vi "main.vi"() -> ()   [LabVIEW 2020]
uses:
  Global 1.vi
  <extravilib>/ChannelInstances/Lossy Stream-a[.,.](dbl)/Instantiate.vi
  <extravilib>/ChannelInstances/Stream-a[.](dbl)/Instantiate.vi
  <extravilib>/ChannelInstances/Lossy Stream-a[.](dbl)/Instantiate.vi
  <extravilib>/ChannelInstances/Lossy Stream-a[.](u8)/Instantiate.vi
  <vilib>/MakerHub/LINX/Public/Utilities/Open Local.vi
  <extravilib>/ChannelInstances/Stream-a[.,.](dbl)/Instantiate.vi
  <vilib>/MakerHub/LINX/LMH-LINX.lvlib
panel:
  out "Main Loop":i32
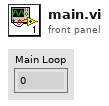
[diagram p1: front panel]
types:
  T1 = enum16{"open", "open or create", "create or replace", "create", "open (read-only)"}
  T2 = typedef "LMH-LINX.lvlib/LINX Ref.ctl" = cluster{"IO":T3, "Interface":T4, "LINX Device Config":T5}
  T3 = typedef "LMH-LINX.lvlib/Platform.ctl" = enum16{"Remote", "Local"}
  T4 = typedef "LMH-LINX.lvlib/Interface.ctl" = enum16{"Serial", "TCP"}
  T5 = typedef "LMH-LINX.lvlib/Device.lvlib/LINX Device Config.ctl" = cluster{"Interface":T4, "COM Port":refnum<visa-resource-name>, "TCP Configuration":T6, "Device Family":u8, "Device ID":u8, "Device Name":string, "TCP Ref":refnum<k5>, "Channels":T7}
  T6 = typedef "LMH-LINX.lvlib/Device.lvlib/TCP Config.ctl" = cluster{"IP Address":string, "Port":u16}
  T7 = typedef "LMH-LINX.lvlib/Channels.ctl" = cluster{"DI":u8[], "DO":u8[], "AI":u8[], "AO":u8[], "PWM":u8[], "QE":u8[], "UART":u8[], "I2C 2":u8[], "SPI":u8[], "CAN":u8[], "Servo":u8[], "AI Ref (V)":dbl, "AI Resolution (Bits)":u8, "AO Ref (V)":dbl, "AO Resolution (Bits)":u8}
  T8 = typedef "Lossy Stream-a[.](u8).lvlib/)Channel.ctl" = refnum<queue>
  T9 = typedef "Lossy Stream-a[.](dbl).lvlib/)Channel.ctl" = refnum<queue>
  T10 = typedef "Stream-a[.](dbl).lvlib/)Channel.ctl" = refnum<queue>
  T11 = typedef "Lossy Stream-a[.,.](dbl).lvlib/)Channel.ctl" = refnum<queue>
  T12 = cluster{"error out":errorcluster, "Error Out":errorcluster, "error out":errorcluster, "error out":errorcluster, "error out":errorcluster}
  T13 = typedef "Stream-a[.,.](dbl).lvlib/)Channel.ctl" = refnum<queue>
  T14 = cluster{"error out":errorcluster, "error out":errorcluster, "Error Out":errorcluster, "error out":errorcluster, "error out":errorcluster, "error out":errorcluster, "error out":errorcluster, "error out":errorcluster}
  T15 = cluster{"Hyperparameters":cluster{"Kernel Type":string, "Alpha (idx)":dbl[][], "Training (idx)":dbl[][], "Label (idx)":dbl[][], "w":dbl[][], "b":dbl, "Performance":cluster{"True Negatives":i32, "False Negatives":i32, "True Positives":i32, "False Positives":i32, "Accuracy":dbl, "F Score":dbl, "Precision":dbl}, "gamma_opt":dbl, "C_opt":dbl}, i32, dbl, "Data Buffer":dbl[][]}
  T16 = cluster{"Kernel Type":string, "Alpha (idx)":dbl[][], "Training (idx)":dbl[][], "Label (idx)":dbl[][], "w":dbl[][], "b":dbl, "Performance":cluster{"True Negatives":i32, "False Negatives":i32, "True Positives":i32, "False Positives":i32, "Accuracy":dbl, "F Score":dbl, "Precision":dbl}, "gamma_opt":dbl, "C_opt":dbl}
  T17 = cluster{"error out":errorcluster, "error out":errorcluster, "Error Out":errorcluster, "error out":errorcluster, "error out":errorcluster, "error out":errorcluster, "error out":errorcluster, "error out":errorcluster, "error out":errorcluster, "error out":errorcluster}
  T18 = cluster{"Kernel Type":string, "Alpha (idx)":dbl[][], "Training (idx)":dbl[][], "Label (idx)":dbl[][], "w":dbl[][], "b":dbl, "Performance":cluster{"True Negatives":i32, "False Negatives":i32, "True Positives":i32, "False Positives":i32, "Accuracy":dbl, "F Score":dbl, "F Score 2":dbl}, "gamma_opt":dbl, "C_opt":dbl}
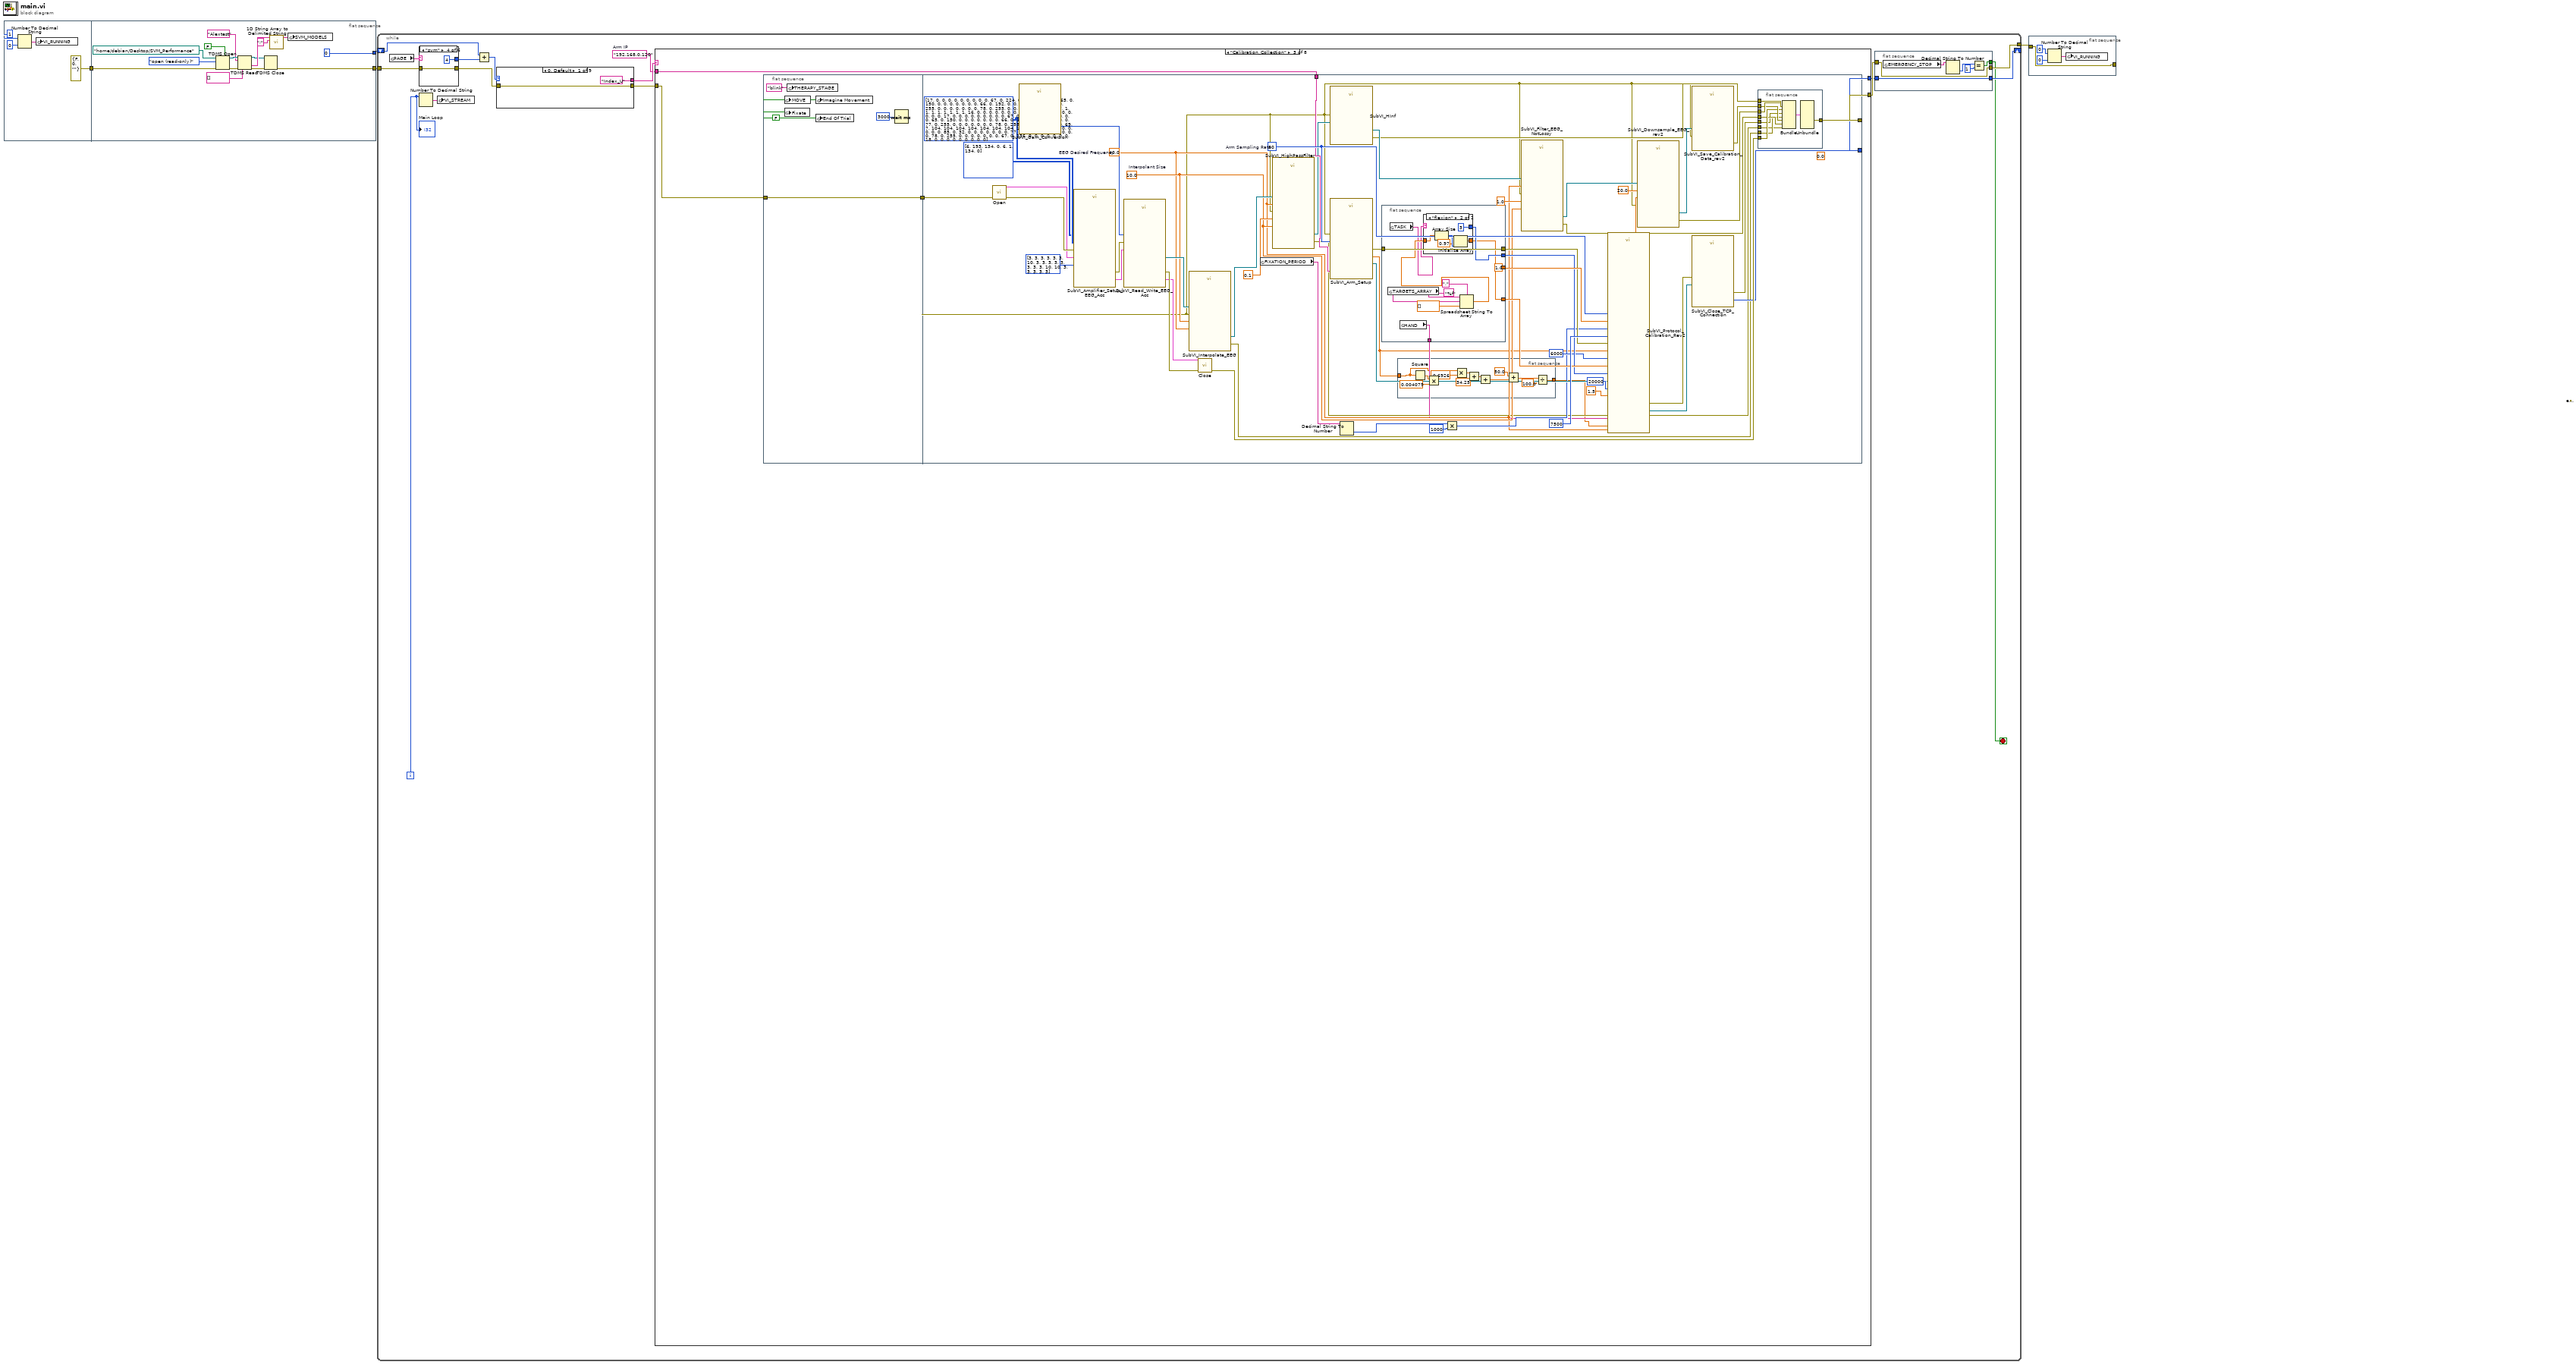
[diagram p0: block diagram]
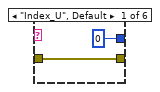
[diagram p2: hidden frame]
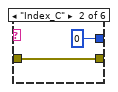
[diagram p3: hidden frame]
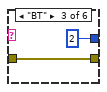
[diagram p4: hidden frame]
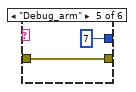
[diagram p5: hidden frame]
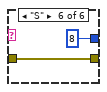
[diagram p6: hidden frame]
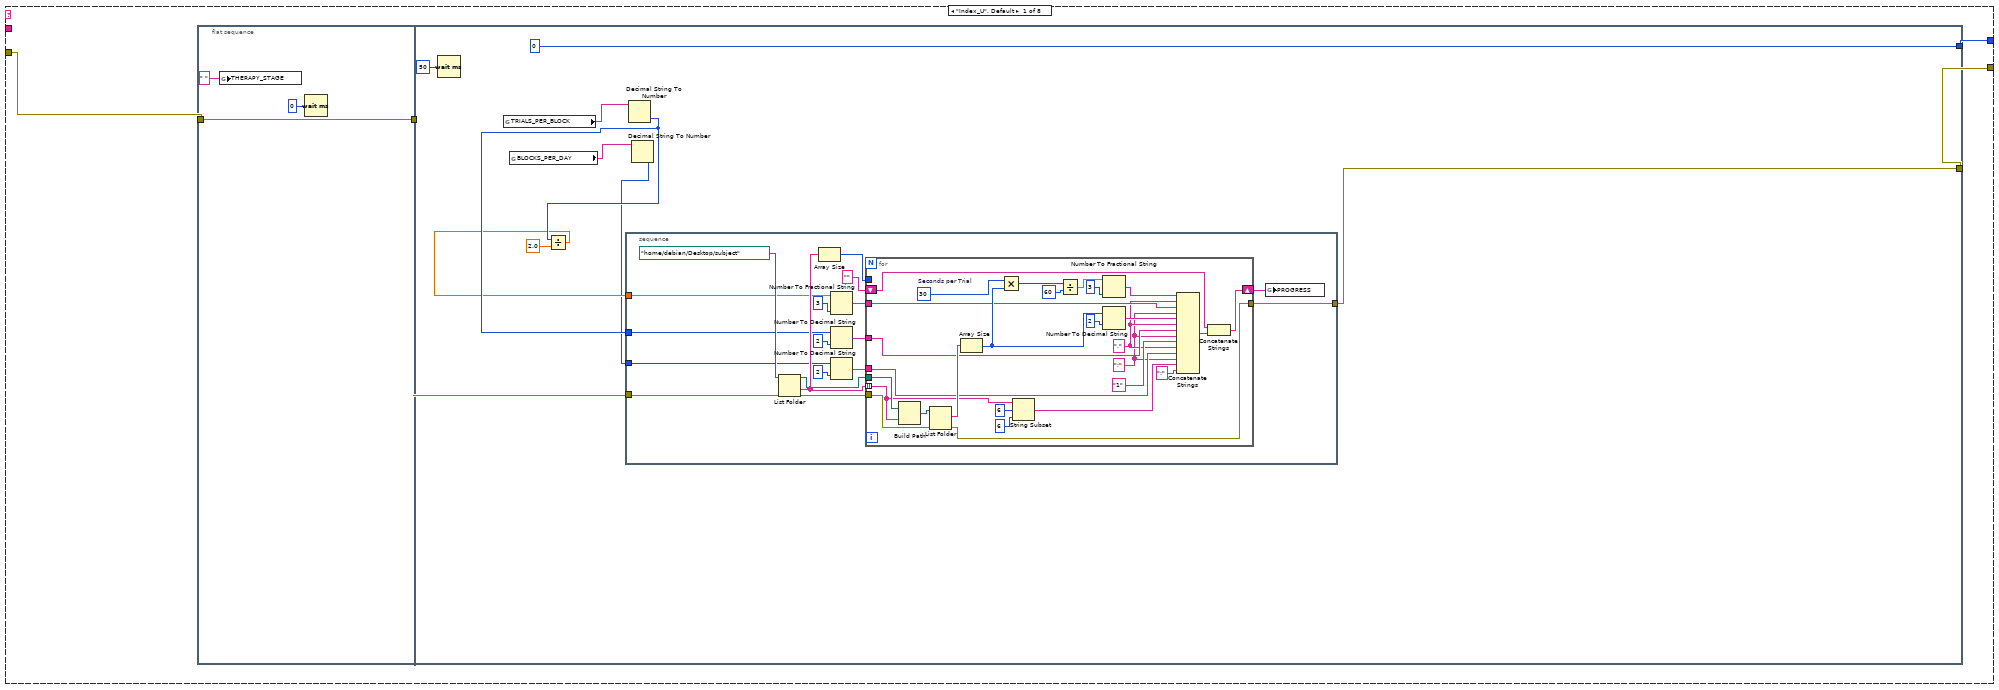
[diagram p7: hidden frame]
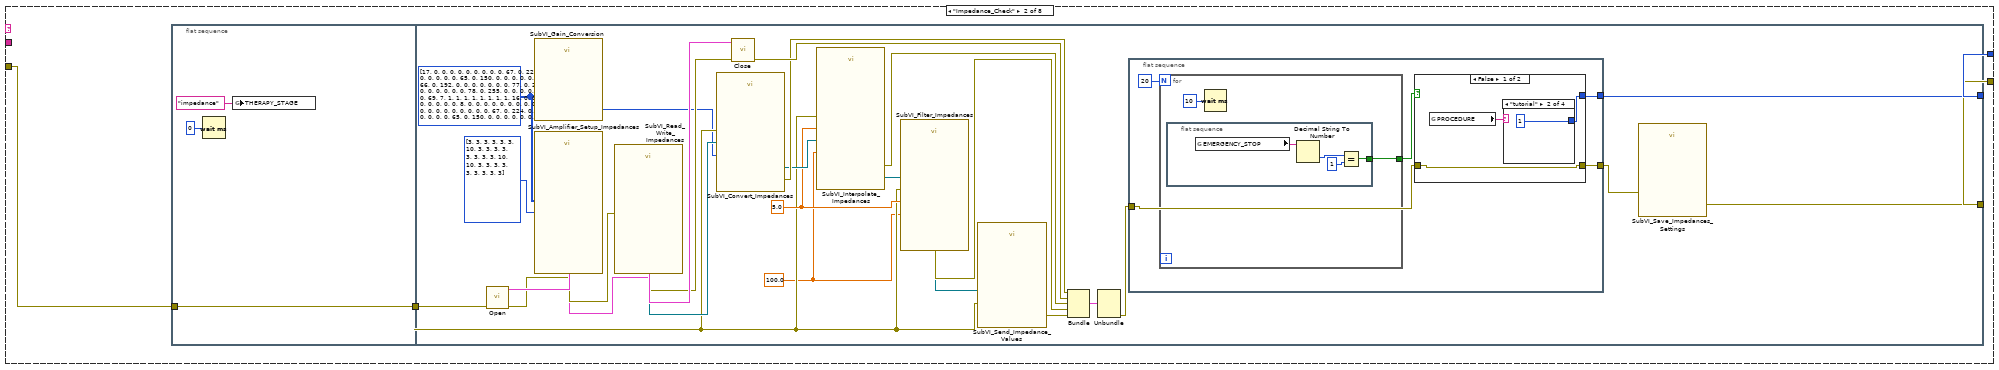
[diagram p8: hidden frame]
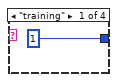
[diagram p9: hidden frame]
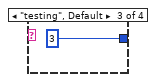
[diagram p10: hidden frame]
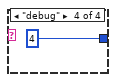
[diagram p11: hidden frame]
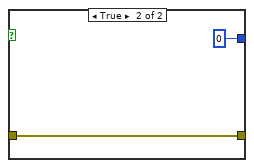
[diagram p12: hidden frame]
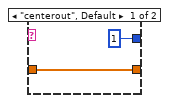
[diagram p13: hidden frame]
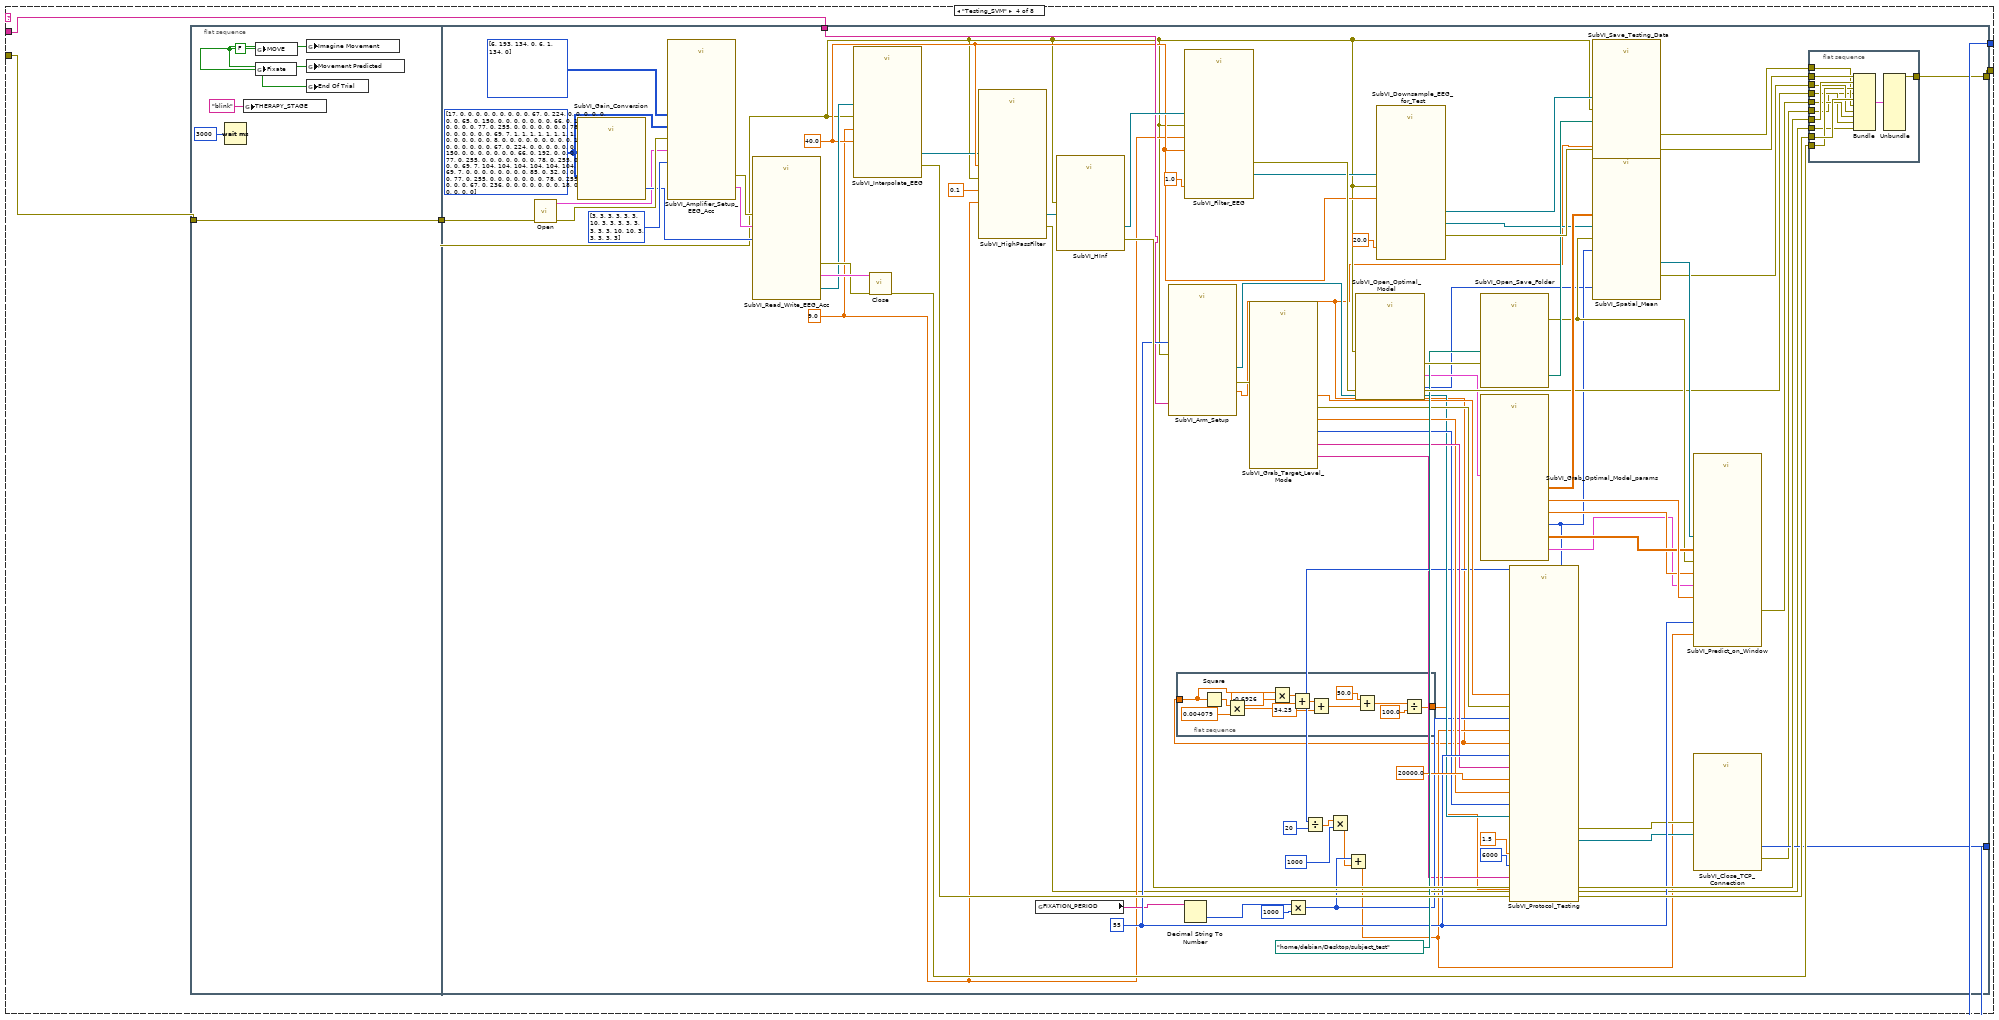
[diagram p14: hidden frame]
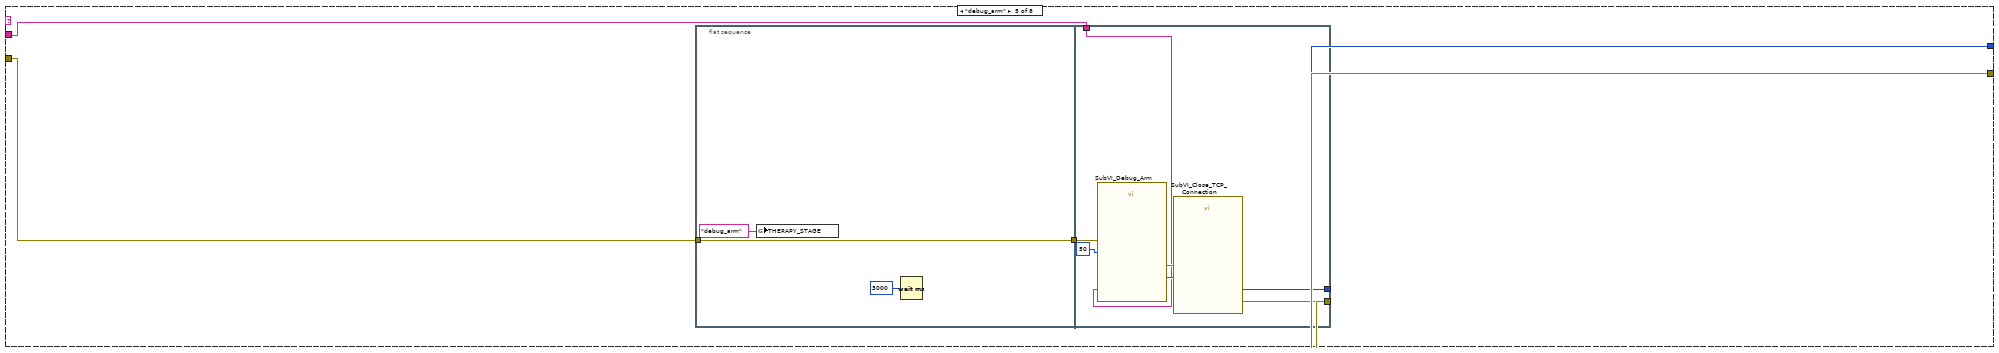
[diagram p15: hidden frame]
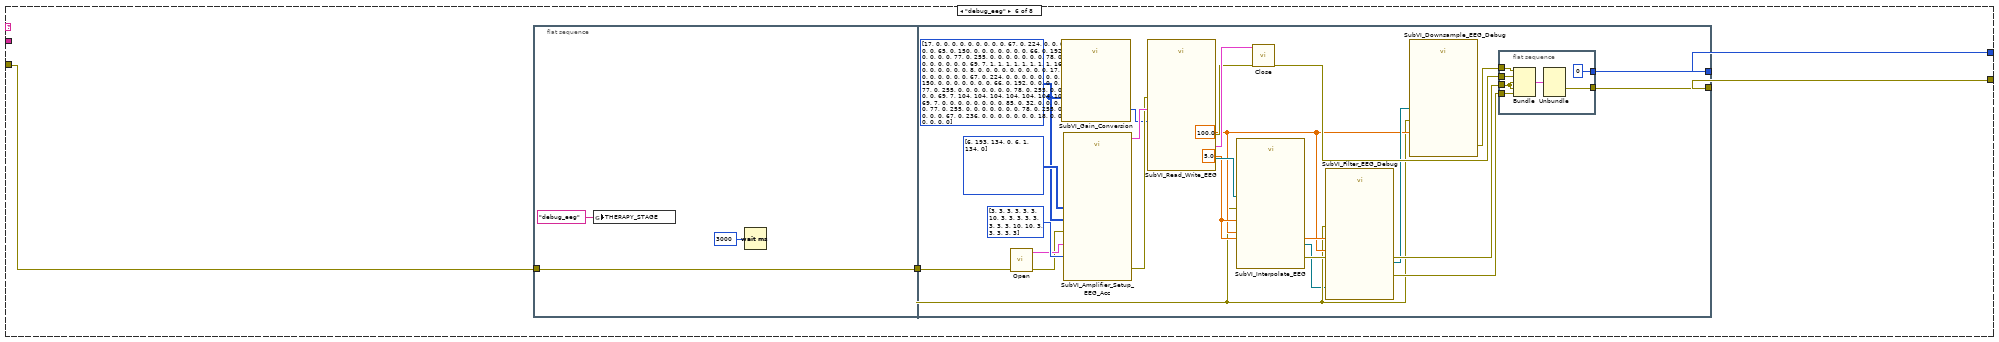
[diagram p16: hidden frame]
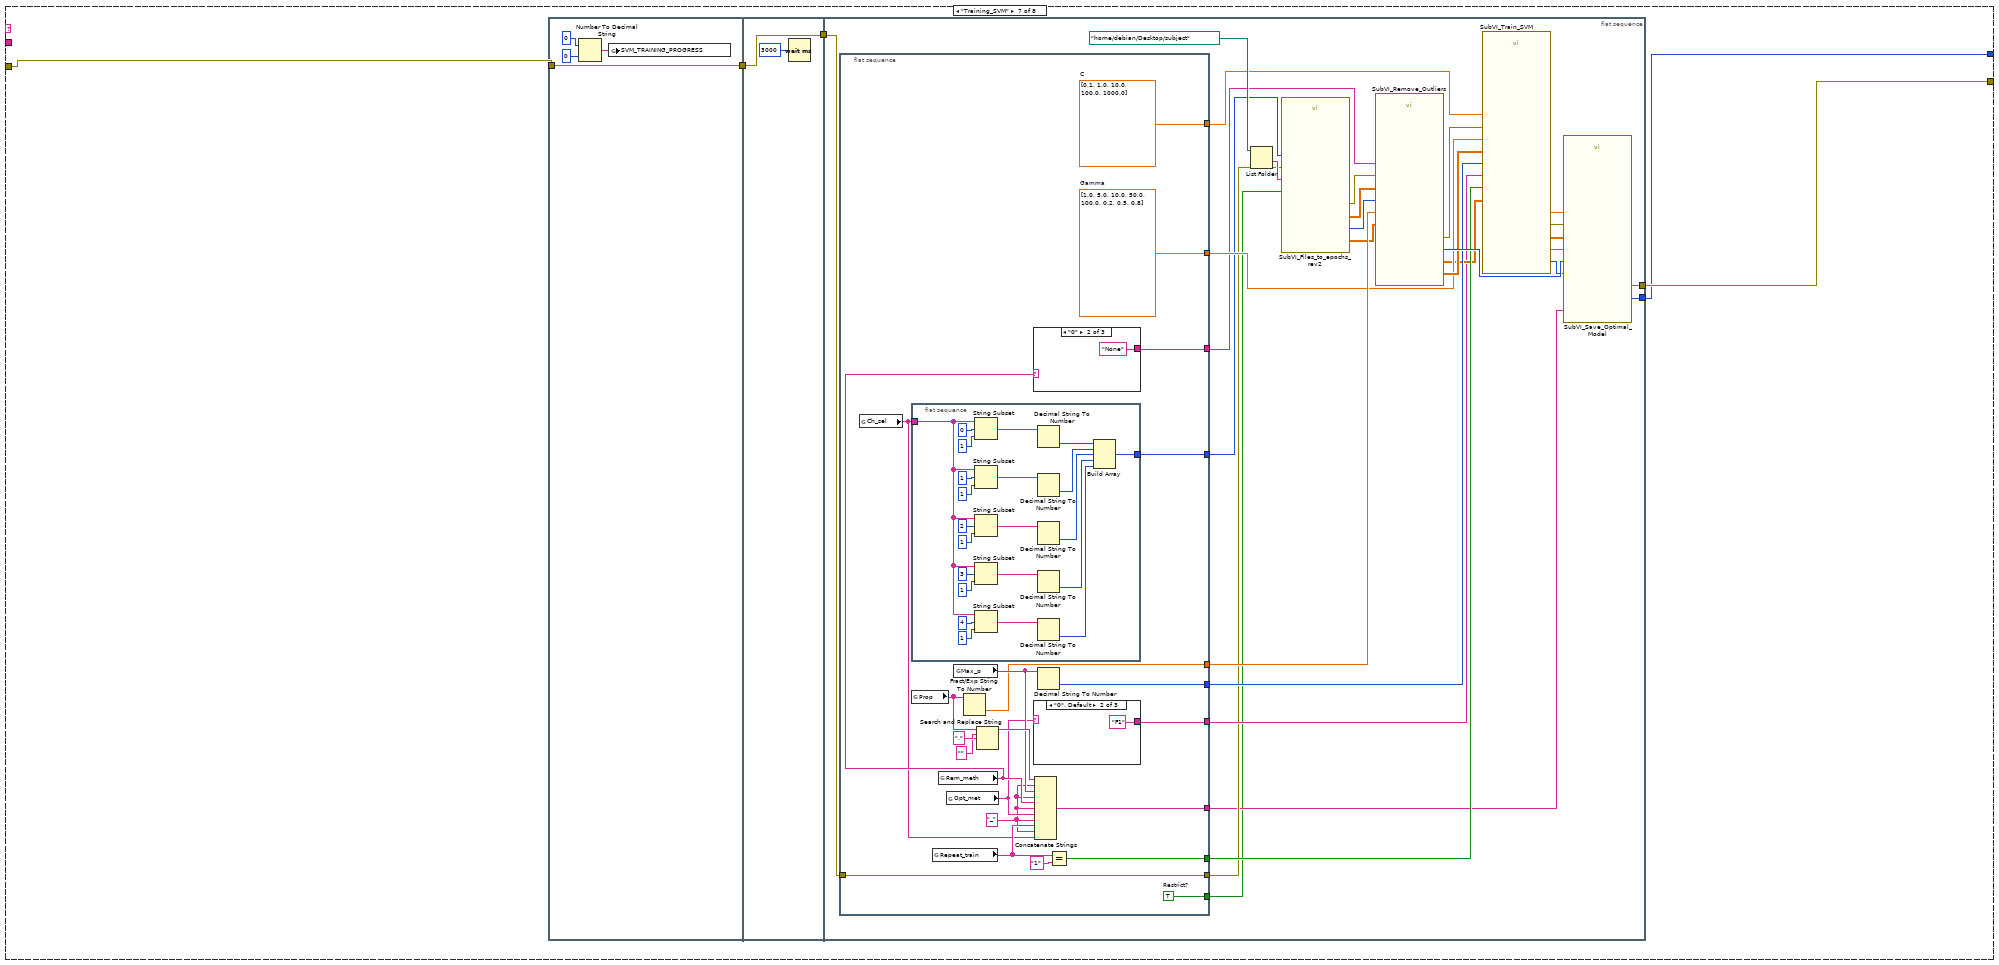
[diagram p17: hidden frame]
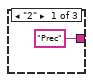
[diagram p18: hidden frame]
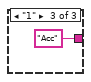
[diagram p19: hidden frame]
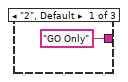
[diagram p20: hidden frame]
diagram:
  (unwired) errorcluster {"status"=FALSE, "code"=0, "source"=""} ("error in (no error)")
  n1 = flat-sequence {
    tunnel: [errorcluster {"status"=FALSE, "code"=0, "source"=""} ("error in (no error)")] -> w2
    tunnel: w2 -> [w13]
    tunnel: [w10] -> w4
    tunnel: [0] -> w1
    frame #0 {
      n2 = Number To Decimal String(number=1, width (-)=i16 0) -> (decimal integer string=w8:string)
      n3 = global write "Global 1.vi" "VI_RUNNING"(w8) -> ()
    }
    frame #1 {
      n4 = TDMS Open(5:FALSE ("create index file? (T)"), 8:w13, 10:T1."open (read-only)" ("operation (0:open)"), 11:path "/home/debian/Desktop/SVM_Performance" ("base path")) -> (0:w18:errorcluster, 3:w19:refnum<k34>)  [unwired: 3 in]
      n5 = TDMS Read(0:w19, 5:"Alextest" ("group name in (Untitled)"), 11:w18, 12:string[] []) -> (4:w21:refnum<k34>, 10:w22:string[], 15:w20:errorcluster)  [unwired: 4 in, 3 out]
      n6 = TDMS Close(8:w20, 11:w21) -> (0:w10:errorcluster)  [unwired: 1 out]
      n7 = call <vilib>:"1D String Array to Delimited String.vi"("delimiter"=";", "string array"=w22) -> ("delimited string"=w23:string)  [unwired: 9 in]
      n8 = global write "Global 1.vi" "SVM_MODELS"(w23) -> ()
    }
  }
  n9 = while {
    tunnel: w4 -> [w35]
    tunnel: [w27] -> w3
    shift-right: [w28] -> _
    shift-left: w1 -> [w33]
    i -> [w31]
    stop <- w25 stop-if-true
    w24 = "192.168.0.120"  # Arm IP
    n10 = global read "Global 1.vi" "PAGE"() -> (w32:string)
    n11 = case shown="\"svm\"" w32 {
      tunnel: [0 0 2 4 7 8] -> w39
      tunnel: [w46 w48 w50 w53 w54 w56] -> w36
      tunnel: w35 -> [w46 w48 w50 w53 w54 w56]
      frame "Index_U", Default {
      }
      frame "Index_C" {
      }
      frame "BT" {
      }
      frame "svm" {
      }
      frame "Debug_arm" {
      }
      frame "S" {
      }
    }
    n12 = Number To Decimal String(number=w31) -> (decimal integer string=w30:string)  [unwired: 1 in]
    n13 = global write "Global 1.vi" "VI_STREAM"(w30) -> ()
    n14 = Add(x=w33, y=w39) -> (x+y=w38:i32)
    n15 = case shown="0, Default" w38 {
      tunnel: ["Index_U" "Index_C" "Impedance_Check" "Calibration_Collection" "Training_SVM" "Testing_SVM" "debug_eeg" "debug_arm" "Survey"] -> w37
      tunnel: w36 -> [w537 w539 w542 w545 w548 w551 w554 w557 w559]
      tunnel: [w537 w539 w542 w545 w548 w551 w554 w557 w559] -> w34
      frame 0, Default {
      }
      frame 1 {
      }
      frame 2 {
        n16 = global write "Global 1.vi" "THERAPY_STAGE"("impedance" ("THERAPY_STAGE")) -> ()
      }
      frame 3 {
        n17 = global write "Global 1.vi" "THERAPY_STAGE"(" " ("THERAPY_STAGE")) -> ()
      }
      frame 4 {
        n18 = global write "Global 1.vi" "THERAPY_STAGE"(" " ("THERAPY_STAGE")) -> ()
      }
      frame 5 {
        n19 = global write "Global 1.vi" "THERAPY_STAGE"(" " ("THERAPY_STAGE")) -> ()
      }
      frame 6 {
        n20 = global write "Global 1.vi" "THERAPY_STAGE"(" " ("THERAPY_STAGE")) -> ()
      }
      frame 7 {
        n21 = global write "Global 1.vi" "THERAPY_STAGE"(" " ("THERAPY_STAGE")) -> ()
      }
      frame 8 {
      }
    }
    n22 = case shown="\"Calibration_Collection\"" w37 {
      tunnel: [w59 w123 w177 w281 w387 w402 w439 w528] -> w26
      tunnel: w34 -> [w61 w124 w176 w279 w389 w401 w438 w530]
      tunnel: [w60 w121 w178 w280 w388 w403 w440 w529] -> w29
      tunnel: w24 -> [_ _ w175 w277 w385 _ _ _]
      frame "Index_U", Default {
        n23 = flat-sequence {
          tunnel: w61 -> [w64]
          tunnel: [w64] -> w58
          tunnel: [w71] -> w60
          tunnel: [0 ("Tab Select")] -> w59
          tunnel: w58 -> [w72]
          frame #0 {
            n24 = global write "Global 1.vi" "THERAPY_STAGE"(" " ("THERAPY_STAGE")) -> ()
            n25 = Wait (ms)(milliseconds to wait=u32 0) -> ()  [unwired: 1 out]
          }
          frame #1 {
            n26 = Wait (ms)(milliseconds to wait=u32 50) -> ()  [unwired: 1 out]
            n27 = global read "Global 1.vi" "TRIALS_PER_BLOCK"() -> (w69:string)
            n28 = global read "Global 1.vi" "BLOCKS_PER_DAY"() -> (w70:string)
            n29 = Decimal String To Number(string=w69) -> (number=w67:i32)  [unwired: 2 in, 1 out]
            n30 = Divide(x=w67, y=2.0) -> (x/y=w66:dbl)
            n31 = Decimal String To Number(string=w70) -> (number=w65:i32)  [unwired: 2 in, 1 out]
            n32 = stacked-sequence {
              tunnel: w72 -> [w92]
              tunnel: w66 -> [w80]
              tunnel: w65 -> [w82]
              tunnel: w67 -> [w81]
              tunnel: [w75] -> w71
              frame #0 {
                n33 = List Folder(path=path "/home/debian/Desktop/subject" ("base path"), error in=w92) -> (path out=w90:path, folder names=w88:string[], error out=w89:errorcluster)  [unwired: 2 in, 1 out]
                n34 = Array Size(array=w88) -> (size(s)=w87:i32)
                n35 = Number To Fractional String(number=w80, precision (6)=i16 3) -> (F-format string=w79:string)  [unwired: 2 in]
                n36 = Number To Decimal String(number=w81, width (-)=i16 2) -> (decimal integer string=w78:string)
                n37 = Number To Decimal String(number=w82, width (-)=i16 2) -> (decimal integer string=w77:string)
                n38 = for {
                  tunnel: w88 -> [w96] mode=indexing
                  tunnel: w90 -> [w120]
                  tunnel: w89 -> [w118]
                  tunnel: [w117] -> w75
                  tunnel: w87 -> [_]
                  shift-right: [w115] -> w76
                  shift-left: "" -> [w116]
                  tunnel: w79 -> [w104]
                  tunnel: w78 -> [w102]
                  tunnel: w77 -> [w99]
                  w98 = ";" ("string")
                  w100 = "," ("string")
                  w112 = 30  # Seconds per Trial
                  n39 = Build Path(base path=w120, name or relative path=w96) -> (appended path=w119:path)
                  n40 = List Folder(path=w119, error in=w118) -> (filenames=w114:string[], error out=w117:errorcluster)  [unwired: 2 in, 2 out]
                  n41 = Array Size(array=w114) -> (size(s)=w107:i32)
                  n42 = Multiply(x=w112, y=w107) -> (x*y=w111:i32)
                  n43 = String Subset(string=w96, offset (0)=6, length (rest)=6 ("length (rest)")) -> (substring=w93:string)
                  n44 = Divide(x=w111, y=60) -> (x/y=w108:dbl)
                  n45 = Number To Fractional String(number=w108, precision (6)=i16 3) -> (F-format string=w106:string)  [unwired: 2 in]
                  n46 = Number To Decimal String(number=w107, width (-)=i16 2) -> (decimal integer string=w103:string)
                  n47 = Concatenate Strings(w106, w100, w104, w98, w103, w100, w102, w98, "1" ("string"), w100, w99, w98, w93, ":" ("string")) -> (w105:string)
                  n48 = Concatenate Strings(w116, w105) -> (w115:string)
                }
                n49 = global write "Global 1.vi" "PROGRESS"(w76) -> ()
              }
            }
          }
        }
      }
      frame "Impedance_Check" {
        n50 = flat-sequence {
          tunnel: w124 -> [w127]
          tunnel: [w127] -> w122
          tunnel: [w134] -> w123
          tunnel: w122 -> [w136]
          tunnel: [w128] -> w121
          frame #0 {
            n51 = Wait (ms)(milliseconds to wait=u32 0) -> ()  [unwired: 1 out]
            n52 = global write "Global 1.vi" "THERAPY_STAGE"("impedance" ("THERAPY_STAGE")) -> ()
          }
          frame #1 {
            w144 = 5.0 ("Resampling rate")
            w135 = 100.0 ("Resampling rate")
            w131 = u8[][] [[17, 0, 0, 0, 0, 0, 0, 0, 0, 0], [67, 0, 224, 0, 0, 0, 0, 0, 0, 0], [65, 0, 150, 0, 0, 0, 0, 0, 0, 0], [66, 0, 192, 0, 0, 0, 0, 0, 0, 0], [77, 0, 255, 0, 0, 0, 0, 0, 0, 0], [78, 0, 255, 0, 0, 0, 0, 0, 0, 0], [69, 7, 1, 1, 1, 1, 1, 1, 1, 1], [16, 0, 0, 0, 0, 0, 0, 0, 0, 0], [8, 0, 0, 0, 0, 0, 0, 0, 0, 0], [17, 0, 0, 0, 0, 0, 0, 0, 0, 0], [67, 0, 224, 0, 0, 0, 0, 0, 0, 0], [65, 0, 150, 0, 0, 0, 0, 0, 0, 0], [66, 0, 192, 0, 0, 0, 0, 0, 0, 0], [77, 0, 255, 0, 0, 0, 0, 0, 0, 0], [78, 0, 255, 0, 0, 0, 0, 0, 0, 0], [69, 7, 104, 104, 104, 104, 104, 104, 104, 104], [69, 7, 0, 0, 0, 0, 0, 0, 0, 0], [85, 0, 32, 0, 0, 0, 0, 0, 0, 0], [77, 0, 255, 0, 0, 0, 0, 0, 0, 0], [78, 0, 255, 0, 0, 0, 0, 0, 0, 0], [66, 0, 208, 0, 0, 0, 0, 0, 0, 0], [67, 0, 228, 0, 0, 0, 0, 0, 0, 0], [68, 0, 2, 0, 0, 0, 0, 0, 0, 0], [79, 0, 255, 0, 0, 0, 0, 0, 0, 0], [80, 0, 0, 0, 0, 0, 0, 0, 0, 0], [18, 0, 0, 0, 0, 0, 0, 0, 0, 0]] ("Data")
            n53 = call-poly <vilib>:"Open.vi"("Error In"=w136) -> ("Error Out"=w132:errorcluster, "LINX Resource"=w151:T2)  [unwired: 8 in, 1 out]
            n54 = call "SubVI_Gain_Conversion.vi"("Amp commands"=w131) -> ("Gain Weights"=w130:i32[])  [unwired: 10 in]
            n55 = call "SubVI_Amplifier_Setup_Impedances.vi"("error in (no error)"=w132, "LINX Resource in"=w151, "Command Row Lenghts"=u8[] [3, 3, 3, 3, 3, 3, 10, 3, 3, 3, 3, 3, 3, 3, 3, 10, 10, 3, 3, 3, 3, 3, 3, 3, 3, 3] ("Data"), "Amplifier Commands"=w131) -> ("error out"=w139:errorcluster, "LINX Resource out"=w138:T2)  [unwired: 6 in]
            n56 = call "SubVI_Read_Write_Impedances.vi"("error in (no error)"=w139, "LINX Resource in"=w138) -> ("error out"=w152:errorcluster, "LINX Resource out"=w153:T2, "Raw Impedances Out"=w150:T8)  [unwired: 7 in]
            n57 = call "SubVI_Convert_Impedances.vi"("error in (no error)"=w136, "Weight Array"=w130, "Raw Impedances in"=w150) -> ("error out"=w148:errorcluster, "Converted Impedances Out"=w147:T9)  [unwired: 7 in]
            n58 = call <vilib>:"Close.vi"("Error In"=w152, "LINX Resource"=w153) -> ("Error Out"=w149:errorcluster)  [unwired: 9 in]
            n59 = call "SubVI_Interpolate_Impedances.vi"("error in (no error)"=w136, "Resampling rate"=w135, "Interpolant Size"=w144, "Raw Impedances In"=w147) -> ("error out"=w146:errorcluster, "Interpolated Impedances Out"=w145:T10)  [unwired: 6 in]
            n60 = call "SubVI_Filter_Impedances.vi"("error in (no error)"=w136, "Resampling rate"=w135, "Interpolant Size"=w144, "Constant Impedances In"=w145) -> ("error out"=w143:errorcluster, "Filtered Impedances Out"=w142:T11)  [unwired: 6 in]
            n61 = call "SubVI_Send_Impedance_Values.vi"("error in (no error)"=w136, "Raw Impedances In"=w142) -> ("error out"=w141:errorcluster)  [unwired: 9 in]
            n62 = Bundle("error out"=w148, "Error Out"=w149, "error out"=w146, "error out"=w143, "error out"=w141) -> (w137:T12)  [unwired: 1 in]
            n63 = Unbundle(w137) -> ("error out"=w133:errorcluster)  [unwired: 4 out]
            n64 = flat-sequence {
              tunnel: [w158] -> w134
              tunnel: w133 -> [w157]
              tunnel: [w156] -> w129
              frame #0 {
                n65 = for {
                  N: 20 -> [_]
                  tunnel: [w159] -> w155
                  n66 = flat-sequence {
                    tunnel: [w161] -> w159
                    frame #0 {
                      n67 = global read "Global 1.vi" "EMERGENCY_STOP"() -> (w162:string)
                      n68 = Decimal String To Number(string=w162) -> (number=w164:i32)  [unwired: 2 in, 1 out]
                      n69 = Equal?(x=w164, y=1) -> (x = y?=w161:bool)
                    }
                  }
                  n70 = Wait (ms)(milliseconds to wait=u32 10) -> ()  [unwired: 1 out]
                }
                n71 = case shown="False" w155 {
                  tunnel: [w167 0 ("Tab Select")] -> w158
                  tunnel: w157 -> [w166 w172]
                  tunnel: [w166 w172] -> w156
                  frame False {
                    n72 = global read "Global 1.vi" "PROCEDURE"() -> (w165:string)
                    n73 = case shown="\"tutorial\"" w165 {
                      tunnel: [1 ("Tab Select") 1 ("Tab Select") 3 ("Tab Select") 4 ("Tab Select")] -> w167
                      frame "training" {
                      }
                      frame "tutorial" {
                      }
                      frame "testing", Default {
                      }
                      frame "debug" {
                      }
                    }
                  }
                  frame True {
                  }
                }
              }
            }
            n74 = call "SubVI_Save_Impedances_Settings.vi"("error in (no error)"=w129) -> ("error out"=w128:errorcluster)  [unwired: 10 in]
          }
        }
      }
      frame "Calibration_Collection" {
        n75 = flat-sequence {
          tunnel: w176 -> [w182]
          tunnel: [w182] -> w174
          tunnel: [w230] -> w178
          tunnel: [w226] -> w177
          tunnel: w174 -> [w187]
          tunnel: w175 -> [w199]
          frame #0 {
            w181 = FALSE
            n76 = global write "Global 1.vi" "MOVE"(w181) -> ()
            n77 = global write "Global 1.vi" "Fixate"(w181) -> ()
            n78 = global write "Global 1.vi" "THERAPY_STAGE"("blink" ("THERAPY_STAGE")) -> ()
            n79 = global write "Global 1.vi" "Imagine Movement"(w181) -> ()
            n80 = global write "Global 1.vi" "End Of Trial"(w181) -> ()
            n81 = Wait (ms)(milliseconds to wait=u32 3000) -> ()  [unwired: 1 out]
          }
          frame #1 {
            (unwired) 0.0 ("EEG Desired Frequency")
            w208 = u32 50  # Arm Sampling Rate
            w223 = u8[][] [[17, 0, 0, 0, 0, 0, 0, 0, 0, 0], [67, 0, 224, 0, 0, 0, 0, 0, 0, 0], [65, 0, 150, 0, 0, 0, 0, 0, 0, 0], [66, 0, 192, 0, 0, 0, 0, 0, 0, 0], [77, 0, 255, 0, 0, 0, 0, 0, 0, 0], [78, 0, 255, 0, 0, 0, 0, 0, 0, 0], [69, 7, 1, 1, 1, 1, 1, 1, 1, 1], [16, 0, 0, 0, 0, 0, 0, 0, 0, 0], [8, 0, 0, 0, 0, 0, 0, 0, 0, 0], [17, 0, 0, 0, 0, 0, 0, 0, 0, 0], [67, 0, 224, 0, 0, 0, 0, 0, 0, 0], [65, 0, 150, 0, 0, 0, 0, 0, 0, 0], [66, 0, 192, 0, 0, 0, 0, 0, 0, 0], [77, 0, 255, 0, 0, 0, 0, 0, 0, 0], [78, 0, 255, 0, 0, 0, 0, 0, 0, 0], [69, 7, 104, 104, 104, 104, 104, 104, 104, 104], [69, 7, 0, 0, 0, 0, 0, 0, 0, 0], [85, 0, 32, 0, 0, 0, 0, 0, 0, 0], [77, 0, 255, 0, 0, 0, 0, 0, 0, 0], [78, 0, 255, 0, 0, 0, 0, 0, 0, 0], [67, 0, 236, 0, 0, 0, 0, 0, 0, 0], [18, 0, 0, 0, 0, 0, 0, 0, 0, 0]] ("Data")
            w191 = 40.0  # EEG Desired Frequency
            w192 = 10.0  # Interpolant Size
            n82 = call-poly <vilib>:"Open.vi"("Error In"=w187) -> ("Error Out"=w220:errorcluster, "LINX Resource"=w219:T2)  [unwired: 8 in, 1 out]
            n83 = call "SubVI_Gain_Conversion.vi"("Amp commands"=w223) -> ("Gain Weights"=w228:i32[])  [unwired: 10 in]
            n84 = call "SubVI_Amplifier_Setup_EEG_Acc.vi"("LINX Resource in"=w219, "error in (no error)"=w220, "Size of Rows for EEG Setup"=u8[] [3, 3, 3, 3, 3, 3, 10, 3, 3, 3, 3, 3, 3, 3, 3, 10, 10, 3, 3, 3, 3, 3] ("Data"), "Amplifier Acc Setup"=u8[][] [[6, 193], [134, 0], [6, 1], [134, 0]] ("Data"), "Amplifier EEG Setup"=w223) -> ("error out"=w217:errorcluster, "LINX Resource out"=w218:T2)  [unwired: 5 in]
            n85 = call "SubVI_Read_Write_EEG_Acc.vi"("error in (no error)"=w217, "Weight Array"=w228, "LINX Resource in"=w218) -> ("error out"=w235:errorcluster, "Raw EEG"=w216:T9, "LINX Resource out"=w225:T2)  [unwired: 5 in, 1 out]
            n86 = call "SubVI_Interpolate_EEG.vi"("error in (no error)"=w187, "Interpolant Size"=w192, "Resampling rate"=w191, "Converted EEG"=w216) -> ("error out"=w215:errorcluster, "EEG"=w193:T10)  [unwired: 6 in]
            n87 = call <vilib>:"Close.vi"("Error In"=w235, "LINX Resource"=w225) -> ("Error Out"=w231:errorcluster)  [unwired: 9 in]
            n88 = global read "Global 1.vi" "FIXATION_PERIOD"() -> (w198:string)
            n89 = call "SubVI_HighPassFilter.vi"("Interpolant Size"=w192, "error in (no error)"=w187, "high cutoff freq"=0.1, "EEG Desired Frequency"=w191, "Channel in"=w193) -> ("error out"=w186:errorcluster, "Channel out"=w190:T10)  [unwired: 5 in]
            n90 = call "SubVI_HInf.vi"("error in (no error)"=w187, "Raw EEG In"=w190) -> ("error out"=w188:errorcluster, "Clean EEG Out"=w189:T13)  [unwired: 8 in]
            n91 = call "SubVI_Arm_Setup.vi"("Arm IP Address"=w199, "error in (no error)"=w187, "Arm Sampling Rate"=w208) -> ("error out"=w214:errorcluster, "Max Position"=w184:dbl, "Arm TCP ID"=w205:refnum<k5>)  [unwired: 6 in]
            n92 = Decimal String To Number(string=w198) -> (number=w196:i32)  [unwired: 2 in, 1 out]
            n93 = flat-sequence {
              tunnel: [w250] -> w207
              tunnel: [1.0] -> w212
              tunnel: [w252] -> w206
              tunnel: w214 -> [w254]
              tunnel: [w254] -> w209
              tunnel: [w253] -> w185
              frame #0 {
                n94 = global read "Global 1.vi" "TARGETS_ARRAY"() -> (w259:string)
                n95 = global read "Global 1.vi" "TASK"() -> (w249:string)
                n96 = global read "Global 1.vi" "HAND"() -> (w253:string)
                n97 = Spreadsheet String To Array(delimiter (Tab)=",", format string="%f", spreadsheet string=w259, array type (2D Dbl)=dbl[] []) -> (array=w251:dbl[])
                n98 = case shown="\"flexion\"" w249 {
                  tunnel: [1 3] -> w252
                  tunnel: w251 -> [w260 w265]
                  tunnel: [w260 w262] -> w250
                  frame "centerout", Default {
                  }
                  frame "flexion" {
                    n99 = Array Size(array=w265) -> (size(s)=w264:i32)
                    n100 = Initialize Array(0.97 ("element"), w264) -> (w262:dbl[])
                  }
                }
              }
            }
            n101 = flat-sequence {
              tunnel: w184 -> [w242]
              tunnel: [w245] -> w183
              frame #0 {
                n102 = Square(x=w242) -> (x^2=w244:dbl)
                n103 = Multiply(x=w244, y=0.004079) -> (x*y=w239:dbl)
                n104 = Multiply(x=w242, y=-0.6926) -> (x*y=w240:dbl)
                n105 = Add(x=w240, y=w239) -> (x+y=w238:dbl)
                n106 = Add(x=w238, y=34.25) -> (x+y=w236:dbl)
                n107 = Add(x=50.0, y=w236) -> (x+y=w247:dbl)
                n108 = Divide(x=w247, y=100.0) -> (x/y=w245:dbl)
              }
            }
            n109 = Multiply(x=w196, y=1000) -> (x*y=w195:i32)
            n110 = call "SubVI_Filter_EEG_NotLossy.vi"("Interpolant Size"=w192, "error in (no error)"=w187, "high cutoff freq"=1.0, "EEG Desired Frequency"=w191, "Channel in"=w189) -> ("error out"=w224:errorcluster, "Channel out"=w229:T13)  [unwired: 5 in]
            n111 = call "SubVI_Protocol_Calibration_Rev2.vi"("TCP Network Connection in"=w205, "ATAN scaler"=1.5 ("y"), "Task"=w206, "Rest Period Length"=6000, "Current Level"=w212, "error in (no error)"=w209, "Total trial length"=20000, "Max Position"=w184, "End of Imagine"=7500, "Target array"=w207, "End of Fixate"=w195, "Arm Sampling Rate"=w208, "MidOut Proportion"=w183, "Arm"=w185) -> ("TCP Network Connection out"=w204:refnum<k5>, "error out"=w203:errorcluster)  [unwired: 4 in]
            n112 = call "SubVI_Downsample_EEG_rev2.vi"("error in (no error)"=w187, "Downsampling Rate"=20.0, "EEG Desired Frequency"=w191, "Channel in"=w229) -> ("error out"=w234:errorcluster, "Channel out"=w233:T10)  [unwired: 6 in]
            n113 = call "SubVI_Save_Calibration_Data_rev2.vi"("error in (no error)"=w187, "Channel in"=w233) -> ("error out"=w232:errorcluster)  [unwired: 9 in]
            n114 = call "SubVI_Close_TCP_Connection.vi"("error in (no error)"=w203, "TCP Network Connection in"=w204) -> ("error out"=w227:errorcluster, "Case to Switch to following Close"=w226:i32)  [unwired: 8 in]
            n115 = flat-sequence {
              tunnel: w188 -> [w276]
              tunnel: w234 -> [w275]
              tunnel: w232 -> [w274]
              tunnel: w231 -> [w272]
              tunnel: [w269] -> w230
              tunnel: w227 -> [w268]
              tunnel: w224 -> [w271]
              tunnel: w215 -> [w270]
              tunnel: w186 -> [w267]
              frame #0 {
                n116 = Bundle("error out"=w275, "error out"=w276, "Error Out"=w272, "error out"=w268, "error out"=w270, "error out"=w274, "error out"=w271, "error out"=w267) -> (w273:T14)  [unwired: 1 in]
                n117 = Unbundle(w273) -> ("error out"=w269:errorcluster)  [unwired: 7 out]
              }
            }
          }
        }
      }
      frame "Testing_SVM" {
        n118 = flat-sequence {
          tunnel: w279 -> [w285]
          tunnel: [w285] -> w278
          tunnel: [w325] -> w281
          tunnel: [w358] -> w280
          tunnel: w278 -> [w300]
          tunnel: w277 -> [w311]
          frame #0 {
            w283 = FALSE
            n119 = Wait (ms)(milliseconds to wait=u32 3000) -> ()  [unwired: 1 out]
            n120 = global write "Global 1.vi" "THERAPY_STAGE"("blink" ("THERAPY_STAGE")) -> ()
            n121 = global write "Global 1.vi" "MOVE"(w283) -> ()
            n122 = global write "Global 1.vi" "Fixate"(w283) -> ()
            n123 = global write "Global 1.vi" "Imagine Movement"(w283) -> ()
            n124 = global write "Global 1.vi" "Movement Predicted"(w283) -> ()
            n125 = global write "Global 1.vi" "End Of Trial"(w283) -> ()
          }
          frame #1 {
            w318 = u32 55 ("milliseconds to wait")
            w331 = u8[][] [[17, 0, 0, 0, 0, 0, 0, 0, 0, 0], [67, 0, 224, 0, 0, 0, 0, 0, 0, 0], [65, 0, 150, 0, 0, 0, 0, 0, 0, 0], [66, 0, 192, 0, 0, 0, 0, 0, 0, 0], [77, 0, 255, 0, 0, 0, 0, 0, 0, 0], [78, 0, 255, 0, 0, 0, 0, 0, 0, 0], [69, 7, 1, 1, 1, 1, 1, 1, 1, 1], [16, 0, 0, 0, 0, 0, 0, 0, 0, 0], [8, 0, 0, 0, 0, 0, 0, 0, 0, 0], [17, 0, 0, 0, 0, 0, 0, 0, 0, 0], [67, 0, 224, 0, 0, 0, 0, 0, 0, 0], [65, 0, 150, 0, 0, 0, 0, 0, 0, 0], [66, 0, 192, 0, 0, 0, 0, 0, 0, 0], [77, 0, 255, 0, 0, 0, 0, 0, 0, 0], [78, 0, 255, 0, 0, 0, 0, 0, 0, 0], [69, 7, 104, 104, 104, 104, 104, 104, 104, 104], [69, 7, 0, 0, 0, 0, 0, 0, 0, 0], [85, 0, 32, 0, 0, 0, 0, 0, 0, 0], [77, 0, 255, 0, 0, 0, 0, 0, 0, 0], [78, 0, 255, 0, 0, 0, 0, 0, 0, 0], [67, 0, 236, 0, 0, 0, 0, 0, 0, 0], [18, 0, 0, 0, 0, 0, 0, 0, 0, 0]] ("Data")
            w305 = 40.0 ("Resampling rate")
            w303 = 9.0 ("Raw Samples")
            n126 = call-poly <vilib>:"Open.vi"("Error In"=w300) -> ("Error Out"=w342:errorcluster, "LINX Resource"=w329:T2)  [unwired: 8 in, 1 out]
            n127 = call "SubVI_Gain_Conversion.vi"("Amp commands"=w331) -> ("Gain Weights"=w330:i32[])  [unwired: 10 in]
            n128 = call "SubVI_Amplifier_Setup_EEG_Acc.vi"("LINX Resource in"=w329, "error in (no error)"=w342, "Size of Rows for EEG Setup"=u8[] [3, 3, 3, 3, 3, 3, 10, 3, 3, 3, 3, 3, 3, 3, 3, 10, 10, 3, 3, 3, 3, 3] ("Data"), "Amplifier Acc Setup"=u8[][] [[6, 193], [134, 0], [6, 1], [134, 0]] ("Data"), "Amplifier EEG Setup"=w331) -> ("error out"=w340:errorcluster, "LINX Resource out"=w341:T2)  [unwired: 5 in]
            n129 = call "SubVI_Read_Write_EEG_Acc.vi"("error in (no error)"=w340, "Weight Array"=w330, "LINX Resource in"=w341) -> ("error out"=w338:errorcluster, "Raw EEG"=w337:T9, "LINX Resource out"=w339:T2)  [unwired: 5 in, 1 out]
            n130 = call "SubVI_Interpolate_EEG.vi"("error in (no error)"=w300, "Interpolant Size"=w303, "Resampling rate"=w305, "Converted EEG"=w337) -> ("error out"=w336:errorcluster, "EEG"=w302:T10)  [unwired: 6 in]
            n131 = call <vilib>:"Close.vi"("Error In"=w338, "LINX Resource"=w339) -> ("Error Out"=w327:errorcluster)  [unwired: 9 in]
            n132 = call "SubVI_HighPassFilter.vi"("Interpolant Size"=w303, "error in (no error)"=w300, "high cutoff freq"=0.1, "EEG Desired Frequency"=w305, "Channel in"=w302) -> ("error out"=w299:errorcluster, "Channel out"=w301:T10)  [unwired: 5 in]
            n133 = global read "Global 1.vi" "FIXATION_PERIOD"() -> (w309:string)
            n134 = call "SubVI_HInf.vi"("error in (no error)"=w300, "Raw EEG In"=w301) -> ("error out"=w335:errorcluster, "Clean EEG Out"=w334:T13)  [unwired: 8 in]
            n135 = call "SubVI_Arm_Setup.vi"("Arm IP Address"=w311, "error in (no error)"=w300, "Arm Sampling Rate"=w318) -> ("error out"=w326:errorcluster, "Max Position"=w287:dbl, "Arm TCP ID"=w314:refnum<k5>)  [unwired: 6 in]
            n136 = flat-sequence {
              tunnel: w287 -> [w366]
              tunnel: [w369] -> w286
              frame #0 {
                n137 = Square(x=w366) -> (x^2=w368:dbl)
                n138 = Multiply(x=w368, y=0.004079) -> (x*y=w363:dbl)
                n139 = Multiply(x=w366, y=-0.6926) -> (x*y=w364:dbl)
                n140 = Add(x=w364, y=w363) -> (x+y=w362:dbl)
                n141 = Add(x=w362, y=34.25) -> (x+y=w360:dbl)
                n142 = Add(x=50.0, y=w360) -> (x+y=w371:dbl)
                n143 = Divide(x=w371, y=100.0) -> (x/y=w369:dbl)
              }
            }
            n144 = Decimal String To Number(string=w309) -> (number=w308:i32)  [unwired: 2 in, 1 out]
            n145 = call "SubVI_Filter_EEG.vi"("high cutoff freq"=1.0, "error in (no error)"=w300, "Interpolant Size"=w303, "Resampling rate"=w305, "Clean EEG In"=w334) -> ("error out"=w333:errorcluster, "Filtered EEG Out"=w332:T13)  [unwired: 5 in]
            n146 = call "SubVI_Grab_Target_Level_Mode.vi"("error in (no error)"=w326) -> ("error out"=w320:errorcluster, "Target Array"=w316:dbl[], "Current level"=w321:dbl, "Task"=w315:i32, "HAND"=w288:string, "MODE"=w317:string)  [unwired: 5 in]
            n147 = Multiply(x=w308, y=1000) -> (x*y=w296:i32)
            n148 = call "SubVI_Open_Optimal_Model.vi"("error in (no error)"=w300) -> ("error out"=w347:errorcluster, "Optimal Model Parameters"=w298:T15, "Channel_selection"=w289:i32[])  [unwired: 8 in]
            n149 = call "SubVI_Downsample_EEG_for_Test.vi"("Downsampling rate"=20.0, "error in (no error)"=w300, "Resampling rate"=w305, "Filtered EEG In"=w332) -> ("error out"=w359:errorcluster, "Downsampled EEG for Save Trial"=w356:T10, "Downsampled EEG for Spatial Mean"=w350:T10)  [unwired: 5 in]
            n150 = call "SubVI_Open_Save_Folder.vi"("error in (no error)"=w347, "Save Folder Path"=path "/home/debian/Desktop/subject_test" ("base path")) -> ("error out"=w346:errorcluster, "Resulting Folder Path"=w357:path)  [unwired: 8 in]
            n151 = call "SubVI_Grab_Optimal_Model_params.vi"("Optimal Model Parameters"=w298) -> ("Window Size"=w294:i32, "Zeros Array with window size"=w351:dbl[][], "Covariance Matrix"=w353:dbl[][], "Time Window"=w355:dbl[], "GO Epoch Means"=w352:dbl[], "Hyperparameters"=w297:T16)  [unwired: 5 in]
            n152 = Divide(x=w294, y=20) -> (x/y=w292:dbl)
            n153 = Multiply(x=w292, y=1000) -> (x*y=w290:dbl)
            n154 = Add(x=w296, y=w290) -> (x+y=w295:dbl)
            n155 = call "SubVI_Protocol_Testing.vi"("TCP Network Connection in"=w314, "Current level"=w321, "Rest Period"=6000, "Max Position"=w287, "error in (no error)"=w320, "Target Array"=w316, "milliseconds to wait"=w318, "MidOut Proportion"=w286, "Arm"=w288, "Fixate Limit"=w296, "Task"=w315, "MODE"=w317, "Move Limit"=20000.0, "ATAN Limit"=1.5, "Imagine Minimum Window"=w295) -> ("TCP Network Connection out"=w313:refnum<k5>, "error out"=w312:errorcluster)  [unwired: 3 in]
            n156 = call "SubVI_Save_Testing_Data.vi"("Max_limit"=w287, "error in (no error)"=w300, "Resulting Folder Path"=w357, "Downsampled EEG In"=w356) -> ("error out"=w345:errorcluster)  [unwired: 7 in]
            n157 = call "SubVI_Spatial_Mean.vi"("Channel_select"=w289, "error in (no error)"=w346, "Window Size"=w294, "Time Array"=w351, "Downsampled EEG In"=w350) -> ("error out"=w349:errorcluster, "Spatial Mean Out"=w354:T13)  [unwired: 5 in]
            n158 = call "SubVI_Predict_on_Window.vi"("Protocol waiting period"=w318, "Minimum Imagine Limit"=w295, "Covariance Matrix"=w353, "Time Window"=w355, "error in (no error)"=w346, "GO Epoch Means"=w352, "Hyperparameters"=w297, "Spatial Mean In"=w354) -> ("error out"=w348:errorcluster)  [unwired: 3 in]
            n159 = call "SubVI_Close_TCP_Connection.vi"("error in (no error)"=w312, "TCP Network Connection in"=w313) -> ("error out"=w324:errorcluster, "Case to Switch to following Close"=w325:i32)  [unwired: 8 in]
            n160 = flat-sequence {
              tunnel: w335 -> [w384]
              tunnel: w359 -> [w383]
              tunnel: w336 -> [w382]
              tunnel: [w381] -> w358
              tunnel: w324 -> [w374]
              tunnel: w349 -> [w380]
              tunnel: w327 -> [w379]
              tunnel: w348 -> [w378]
              tunnel: w345 -> [w377]
              tunnel: w333 -> [w376]
              tunnel: w299 -> [w373]
              frame #0 {
                n161 = Bundle("error out"=w383, "error out"=w384, "Error Out"=w379, "error out"=w374, "error out"=w382, "error out"=w377, "error out"=w380, "error out"=w378, "error out"=w376, "error out"=w373) -> (w375:T17)  [unwired: 1 in]
                n162 = Unbundle(w375) -> ("error out"=w381:errorcluster)  [unwired: 9 out]
              }
            }
          }
        }
      }
      frame "debug_arm" {
        n163 = flat-sequence {
          tunnel: w389 -> [w392]
          tunnel: [w392] -> w386
          tunnel: [w394] -> w388
          tunnel: [w395] -> w387
          tunnel: w386 -> [w398]
          tunnel: w385 -> [w393]
          frame #0 {
            n164 = global write "Global 1.vi" "THERAPY_STAGE"("debug_arm" ("THERAPY_STAGE")) -> ()
            n165 = Wait (ms)(milliseconds to wait=u32 3000) -> ()  [unwired: 1 out]
          }
          frame #1 {
            n166 = call "SubVI_Debug_Arm.vi"("Arm IP Address"=w393, "error in (no error)"=w398, "Arm Sampling Rate"=u32 50 ("milliseconds to wait")) -> ("error out"=w396:errorcluster, "TCP Network Connection out"=w397:refnum<k5>)  [unwired: 7 in]
            n167 = call "SubVI_Close_TCP_Connection.vi"("error in (no error)"=w396, "TCP Network Connection in"=w397) -> ("error out"=w394:errorcluster, "Case to Switch to following Close"=w395:i32)  [unwired: 8 in]
          }
        }
      }
      frame "debug_eeg" {
        n168 = flat-sequence {
          tunnel: w401 -> [w406]
          tunnel: [w406] -> w400
          tunnel: [w424] -> w403
          tunnel: [w423] -> w402
          tunnel: w400 -> [w410]
          frame #0 {
            n169 = global write "Global 1.vi" "THERAPY_STAGE"("debug_eeg" ("THERAPY_STAGE")) -> ()
            n170 = Wait (ms)(milliseconds to wait=u32 3000) -> ()  [unwired: 1 out]
          }
          frame #1 {
            w409 = u8[][] [[17, 0, 0, 0, 0, 0, 0, 0, 0, 0], [67, 0, 224, 0, 0, 0, 0, 0, 0, 0], [65, 0, 150, 0, 0, 0, 0, 0, 0, 0], [66, 0, 192, 0, 0, 0, 0, 0, 0, 0], [77, 0, 255, 0, 0, 0, 0, 0, 0, 0], [78, 0, 255, 0, 0, 0, 0, 0, 0, 0], [69, 7, 1, 1, 1, 1, 1, 1, 1, 1], [16, 0, 0, 0, 0, 0, 0, 0, 0, 0], [8, 0, 0, 0, 0, 0, 0, 0, 0, 0], [17, 0, 0, 0, 0, 0, 0, 0, 0, 0], [67, 0, 224, 0, 0, 0, 0, 0, 0, 0], [65, 0, 150, 0, 0, 0, 0, 0, 0, 0], [66, 0, 192, 0, 0, 0, 0, 0, 0, 0], [77, 0, 255, 0, 0, 0, 0, 0, 0, 0], [78, 0, 255, 0, 0, 0, 0, 0, 0, 0], [69, 7, 104, 104, 104, 104, 104, 104, 104, 104], [69, 7, 0, 0, 0, 0, 0, 0, 0, 0], [85, 0, 32, 0, 0, 0, 0, 0, 0, 0], [77, 0, 255, 0, 0, 0, 0, 0, 0, 0], [78, 0, 255, 0, 0, 0, 0, 0, 0, 0], [67, 0, 236, 0, 0, 0, 0, 0, 0, 0], [18, 0, 0, 0, 0, 0, 0, 0, 0, 0]] ("Data")
            w411 = 100.0 ("Resampling rate")
            w414 = 5.0 ("Raw Samples")
            n171 = call-poly <vilib>:"Open.vi"("Error In"=w410) -> ("Error Out"=w417:errorcluster, "LINX Resource"=w419:T2)  [unwired: 8 in, 1 out]
            n172 = call "SubVI_Gain_Conversion.vi"("Amp commands"=w409) -> ("Gain Weights"=w408:i32[])  [unwired: 10 in]
            n173 = call "SubVI_Amplifier_Setup_EEG_Acc.vi"("LINX Resource in"=w419, "error in (no error)"=w417, "Size of Rows for EEG Setup"=u8[] [3, 3, 3, 3, 3, 3, 10, 3, 3, 3, 3, 3, 3, 3, 3, 10, 10, 3, 3, 3, 3, 3] ("Data"), "Amplifier Acc Setup"=u8[][] [[6, 193], [134, 0], [6, 1], [134, 0]] ("Data"), "Amplifier EEG Setup"=w409) -> ("error out"=w416:errorcluster, "LINX Resource out"=w418:T2)  [unwired: 5 in]
            n174 = call "SubVI_Read_Write_EEG.vi"("error in (no error)"=w416, "LINX Resource in"=w418, "Weight Array"=w408) -> ("error out"=w427:errorcluster, "LINX Resource out 2"=w428:T2, "Raw EEG out"=w415:T9)  [unwired: 6 in]
            n175 = call "SubVI_Interpolate_EEG.vi"("error in (no error)"=w410, "Interpolant Size"=w414, "Resampling rate"=w411, "Converted EEG"=w415) -> ("error out"=w413:errorcluster, "EEG"=w407:T10)  [unwired: 6 in]
            n176 = call <vilib>:"Close.vi"("Error In"=w427, "LINX Resource"=w428) -> ("Error Out"=w425:errorcluster)  [unwired: 9 in]
            n177 = call "SubVI_Filter_EEG_Debug.vi"("EEG"=w407, "error in (no error)"=w410, "Resampling rate"=w411, "Interpolant Size"=w414) -> ("error out"=w422:errorcluster, "Filtered EEG Out"=w412:T13)  [unwired: 6 in]
            n178 = call "SubVI_Downsample_EEG_Debug.vi"("error in (no error)"=w410, "Resampling rate"=w411, "Filtered EEG In"=w412) -> ("error out"=w426:errorcluster)  [unwired: 8 in]
            n179 = flat-sequence {
              tunnel: w426 -> [w435]
              tunnel: w425 -> [w430]
              tunnel: w413 -> [w429]
              tunnel: [w433] -> w424
              tunnel: [0 ("Tab Select")] -> w423
              tunnel: w422 -> [w431]
              frame #0 {
                n180 = Bundle("error out"=w435, "Error Out"=w430, "error out"=w429, "error out"=w429, "error out"=w431) -> (w434:T12)  [unwired: 1 in]
                n181 = Unbundle(w434) -> ("error out"=w433:errorcluster)  [unwired: 4 out]
              }
            }
          }
        }
      }
      frame "Training_SVM" {
        n182 = flat-sequence {
          tunnel: w438 -> [w444]
          tunnel: [w444] -> w436
          tunnel: [w446] -> w437
          tunnel: w436 -> [w446]
          tunnel: [w475] -> w440
          tunnel: [w474] -> w439
          tunnel: w437 -> [w458]
          frame #0 {
            n183 = Number To Decimal String(number=0, width (-)=i16 0) -> (decimal integer string=w442:string)
            n184 = global write "Global 1.vi" "SVM_TRAINING_PROGRESS"(w442) -> ()
          }
          frame #1 {
            n185 = Wait (ms)(milliseconds to wait=u32 3000) -> ()  [unwired: 1 out]
          }
          frame #2 {
            n186 = flat-sequence {
              tunnel: [w498] -> w453
              tunnel: [w477] -> w472
              tunnel: [w497] -> w470
              tunnel: [w496] -> w469
              tunnel: [w494] -> w467
              tunnel: [w490] -> w466
              tunnel: [w492] -> w459
              tunnel: w458 -> [w495]
              tunnel: [w495] -> w457
              tunnel: [w493] -> w456
              tunnel: [w489] -> w454
              tunnel: [w488] -> w455
              frame #0 {
                w480 = "_" ("string")
                w498 = TRUE  # Restrict?
                w497 = dbl[] [1.0, 5.0, 10.0, 50.0, 100.0, 0.2, 0.5, 0.8]  # Gamma
                w496 = dbl[] [0.1, 1.0, 10.0, 100.0, 1000.0]  # C
                n187 = global read "Global 1.vi" "Ch_sel"() -> (w479:string)
                n188 = flat-sequence {
                  tunnel: w479 -> [w510]
                  tunnel: [w499] -> w489
                  frame #0 {
                    n189 = String Subset(string=w510, offset (0)=0, length (rest)=1 ("length (rest)")) -> (substring=w509:string)
                    n190 = String Subset(string=w510, offset (0)=1, length (rest)=1 ("length (rest)")) -> (substring=w508:string)
                    n191 = String Subset(string=w510, offset (0)=2, length (rest)=1 ("length (rest)")) -> (substring=w507:string)
                    n192 = String Subset(string=w510, offset (0)=3, length (rest)=1 ("length (rest)")) -> (substring=w506:string)
                    n193 = String Subset(string=w510, offset (0)=4, length (rest)=1 ("length (rest)")) -> (substring=w505:string)
                    n194 = Decimal String To Number(string=w509) -> (number=w504:i32)  [unwired: 2 in, 1 out]
                    n195 = Decimal String To Number(string=w508) -> (number=w503:i32)  [unwired: 2 in, 1 out]
                    n196 = Decimal String To Number(string=w507) -> (number=w502:i32)  [unwired: 2 in, 1 out]
                    n197 = Decimal String To Number(string=w506) -> (number=w501:i32)  [unwired: 2 in, 1 out]
                    n198 = Decimal String To Number(string=w505) -> (number=w500:i32)  [unwired: 2 in, 1 out]
                    n199 = Build Array(w504, w503, w502, w501, w500) -> (w499:i32[])
                  }
                }
                n200 = global read "Global 1.vi" "Prop"() -> (w478:string)
                n201 = global read "Global 1.vi" "Repeat_train"() -> (w481:string)
                n202 = global read "Global 1.vi" "Rem_meth"() -> (w483:string)
                n203 = global read "Global 1.vi" "Opt_met"() -> (w482:string)
                n204 = global read "Global 1.vi" "Max_p"() -> (w484:string)
                n205 = Fract/Exp String To Number(string=w478) -> (number=w477:dbl)  [unwired: 3 in, 1 out]
                n206 = Search and Replace String(input string=w478, search string=".", replace string="" ("replace string (\"\")")) -> (result string=w485:string)  [unwired: 5 in, 3 out]
                n207 = case shown="\"0\"" w483 {
                  tunnel: ["GO Only" "None" "Both"] -> w493
                  frame "2", Default {
                  }
                  frame "0" {
                  }
                  frame "1" {
                  }
                }
                n208 = case shown="\"0\", Default" w482 {
                  tunnel: ["Prec" "F1" "Acc"] -> w492
                  frame "2" {
                  }
                  frame "0", Default {
                  }
                  frame "1" {
                  }
                }
                n209 = Concatenate Strings(w485, w480, w484, w480, w483, w480, w482, w480, w481, w480, w479) -> (w488:string)
                n210 = Decimal String To Number(string=w484) -> (number=w494:i32)  [unwired: 2 in, 1 out]
                n211 = Equal?(x=w481, y="1") -> (x = y?=w490:bool)
              }
            }
            n212 = List Folder(path=path "/home/debian/Desktop/subject" ("base path"), error in=w457) -> (folder names=w452:string[], error out=w451:errorcluster)  [unwired: 2 in, 2 out]
            n213 = call "SubVI_Files_to_epochs_rev2.vi"("Ch_sel"=w454, "error in (no error)"=w451, "Restrict?"=w453, "folder names"=w452) -> ("error out"=w450:errorcluster, "Number of Trials"=w448:i32, "Rest Epochs"=w447:dbl[][], "Go Epochs"=w449:dbl[][])  [unwired: 4 in]
            n214 = call "SubVI_Remove_Outliers.vi"("Type"=w456, "Go Epochs"=w449, "error in (no error)"=w450, "Proportion to delete"=w472, "Rest Epochs"=w447, "Number of Trials"=w448) -> ("error out"=w468:errorcluster, "Rest Epochs"=w465:dbl[][], "Number of Trials"=w473:i32, "Go Epochs"=w471:dbl[][])  [unwired: 2 in]
            n215 = call "SubVI_Train_SVM.vi"("Rest Epochs"=w465, "Repeat training?"=w466, "Go Epochs in"=w471, "Max Passes"=w467, "error in (no error)"=w468, "Gamma"=w470, "C"=w469, "Optimizer\nMetric"=w459) -> ("Go Epochs out"=w462:dbl[][], "Hyperparameters"=w461:T18, "Best (Metric)"=w464:dbl, "Optimum Window Size"=w460:i32, "error out"=w463:errorcluster)  [unwired: 3 in]
            n216 = call "SubVI_Save_Optimal_Model.vi"("Training_settings"=w455, "Optimum Window Size"=w460, "Number of Trials"=w473, "error in (no error)"=w463, "Hyperparameters"=w461, "Go Epochs in"=w462, "Best (Metric)"=w464) -> ("error out"=w475:errorcluster, "Case to Switch to"=w474:i32)  [unwired: 3 in]
          }
        }
      }
      frame "Survey" {
        n217 = flat-sequence {
          tunnel: w530 -> [w532]
          tunnel: [w532] -> w527
          tunnel: [w534] -> w529
          tunnel: [0 ("Case to Switch to")] -> w528
          tunnel: w527 -> [w535]
          frame #0 {
            n218 = Wait (ms)(milliseconds to wait=u32 500) -> ()  [unwired: 1 out]
          }
          frame #1 {
            n219 = call "SubVI_Save_Survey.vi"("error in (no error)"=w535) -> ("error out"=w534:errorcluster)  [unwired: 10 in]
            n220 = Wait (ms)(milliseconds to wait=u32 500) -> ()  [unwired: 1 out]
          }
        }
      }
    }
    n221 = flat-sequence {
      tunnel: [w42] -> w25
      tunnel: w29 -> [w41]
      tunnel: w26 -> [w40]
      tunnel: [w41] -> w27
      tunnel: [w40] -> w28
      frame #0 {
        n222 = global read "Global 1.vi" "EMERGENCY_STOP"() -> (w43:string)
        n223 = Decimal String To Number(string=w43) -> (number=w45:i32)  [unwired: 2 in, 1 out]
        n224 = Equal?(x=w45, y=1) -> (x = y?=w42:bool)
      }
    }
    "Main Loop" <- w31
  }
  n225 = flat-sequence {
    tunnel: [w564] -> _
    tunnel: w3 -> [w564]
    frame #0 {
      n226 = Number To Decimal String(number=0, width (-)=i16 0) -> (decimal integer string=w563:string)
      n227 = global write "Global 1.vi" "VI_RUNNING"(w563) -> ()
    }
  }
